vi "Write port.vi"(8 "Buttons":bool[](array[boolean]), 9 "Write Port":bool, 10 "Expected Response":string, 11 "Command to Send":string) -> (3 "comandos iguales?":bool)   [LabVIEW 2020, in "Test simulado.lvclass"]
uses:
  Test simulado.lvclass
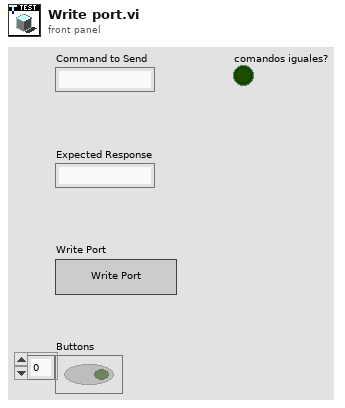
[diagram p1: front panel]
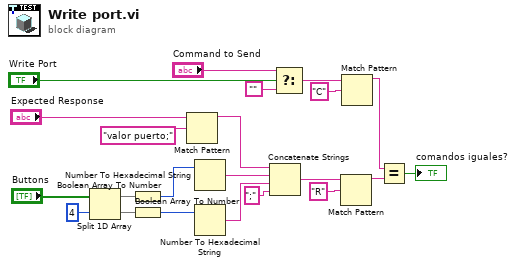
[diagram p0: block diagram]
diagram:
  n1 = Split 1D Array(array="Buttons", index=4) -> (first subarray=w2:bool[], second subarray=w3:bool[])
  n2 = Boolean Array To Number(Boolean array=w2) -> (number=w5:u32)
  n3 = Boolean Array To Number(Boolean array=w3) -> (number=w4:u32)
  n4 = Match Pattern(string="Expected Response", regular expression="valor puerto;") -> (before substring=w8:string)  [unwired: 1 in, 3 out]
  n5 = Number To Hexadecimal String(2:w5) -> (0:w9:string)  [unwired: 1 in]
  n6 = Number To Hexadecimal String(2:w4) -> (0:w10:string)  [unwired: 1 in]
  n7 = Concatenate Strings(w8, w9, w10, ";" ("string")) -> (w18:string)
  n8 = Select(t="Command to Send", s="Write Port", f="") -> (s? t:f=w15:string)
  n9 = Match Pattern(string=w18, regular expression="R") -> (before substring=w20:string)  [unwired: 1 in, 3 out]
  n10 = Match Pattern(string=w15, regular expression="C") -> (before substring=w19:string)  [unwired: 1 in, 3 out]
  n11 = Equal?(x=w19, y=w20) -> (x = y?=→"comandos iguales?":bool)
